vi "Advanced Serial_old.vi"(7 "stop":bool, 8 "read":bool=TRUE, 9 "Write":bool, 11 "string to write":string="*IDN?") -> (0 "RTD-02 (ºC)":sgl format="%0.2f", 1 "RTD-01 (ºC)":sgl format="%0.2f", 2 "vacuo (mBar)":dbl, 3 "P02 (Bar)":dbl, 4 "RTD-chamber (ºC)":sgl format="%0.2f", 5 "P01 (Bar)":dbl, 6 "32bytes":bool)   [LabVIEW 2011]
doc: "The Advanced Serial Read and Write example performs a Serial Port Read, a Serial Port Write, or a combination of these actions while setting some advanced serial features like buffer size, termination characters, and XON/XOFF flow control. The user selects the actions (read or write) on the front panel. If both are selected, the VI will write the data first, read the data and then close the VISA session that is opened to the port. \n\nThe parameters set for the serial port must match the parameters of the connected instrument or device. In this example, the bytes to read parameter specifies the number of bytes that the serial port reads. If there were more bytes at the port than the number specified in bytes to read, those bytes would not be read. Also, if you specify to read more bytes than the number of bytes actually read, you might receive a timeout error message.\n\nINSTRUCTIONS:\n1) Select the serial resource and configuration parameters (baud rate, data bits, parity, stop bits, flow control).\n2) Termination character can be enabled and set. Also, set the required input buffer size prior to running the example.\n3) Select the operations to be performed. \n4) Connect the serial port to your device. If no device is available, perform a loopback test by doing one of the following. Short pins 2 and 3 on a RS-232 cable or short pin 4 to pin 8 and pin 5 to pin 9 on a RS-485/422 cable. \n5) Run the VI to see the data read. (The \"read string\" will match the \"string to write\" if a loopback test was performed.)\n\nThis example exposes several advanced features that you may need for your application. Not all applications need all the features shown in this example. The input buffer size is likely an important setting that you want to control in your application. This example expands upon the flow control option for XON and XOFF, allowing the user to choose those control characters. The timeout parameter has been brought to the front panel so a user can specify the time period the VISA Read will wait for the number of bytes to read before timing out. Also, the user has several controls for the termination character, which is discussed later.\n\nNote that you can press the write and read buttons and change the bytes to read parameters on the fly, while the example is running. However, you must stop the example to change the other configuration parameters after the example has started running, and then run again.\n\nSet the I/O buffer size slightly higher the amount of data you expect to receive. This is very important for applications that don't use flow control, as you may lose characters if the receive buffer overflows.\n\nSetting the timeout period ensures that the operation returns with a timeout error if the operation cannot be performed in the specified time period. \n\nSome devices require a termination character in order to identify the end of command strings. Some devices send a termination character to signify the end of data to be read. \n\nThis example shows how you can end the Read operation once a termination character is detected in the buffer and/or append a termination character at the end of the Write data. To enable the Read to end on a termination character, use the VISA Configure Serial Port or use the VISA Properties Serial End Mode for Reads, Termination Character Enable, and Termination Character. To end the Write with a termination character, use the VISA Properties Serial End Mode for Writes, the Send End Enable, and Termination Character. In this example, the same termination character is used for both the Read and the Write. You can specify two different characters for your application, if desired.\n\nYour application may require specific characters for the XON/XOFF Flow Control. You can specify these characters with the VISA Properties Flow Control XOFF Character and Flow Control XON Character. Note that if the standard XON and XOFF characters are used, then decimal 17 and 19 are unavailable for data values. Remember that using flow control and setting an adequate buffer size allow you to prevent buffer overflows."
uses:
  <vilib>/Instr/_visa.llb/VISA Configure Serial Port (Instr).vi
panel:
  out "actual bytes read":u32
  in  "bytes to read":u32=1000
  out "read string":string
  in  "flow control":u16(ring) items=["None"=0, "XON/XOFF"=1, "RTS/CTS"=2, "DTR/DSR"=4]
  in  "buffer size":u32=4096
  in  "XOFF Character":u8=19 format="%.0x"
  in  "XON Character":u8=17 format="%.0x"
  in  "termination char\n(0xA = '\\n' = LF)":u8=10 format="%.0x"
  in  "timeout (ms)":u32=10000
  in  "parity":u16(ring) items=["None", "Odd", "Even", "Mark", "Space"]
  in  "data bits":u16=8 min=5 max=8 step=1
  in  "stop bits":u16(ring)=10 items=["1.0"=10, "1.5"=15, "2.0"=20]
  out "baud rate":u32=9600
  in  "VISA resource name":refnum<visa-resource-name>="COM1"
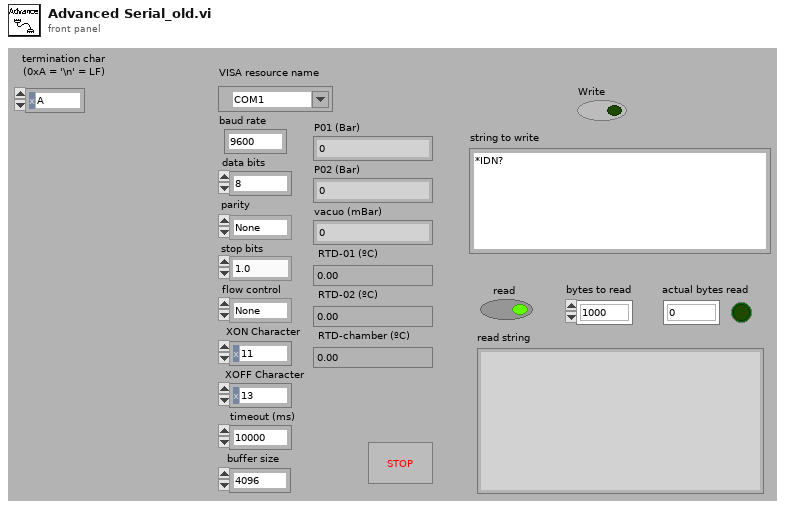
[diagram p1: front panel]
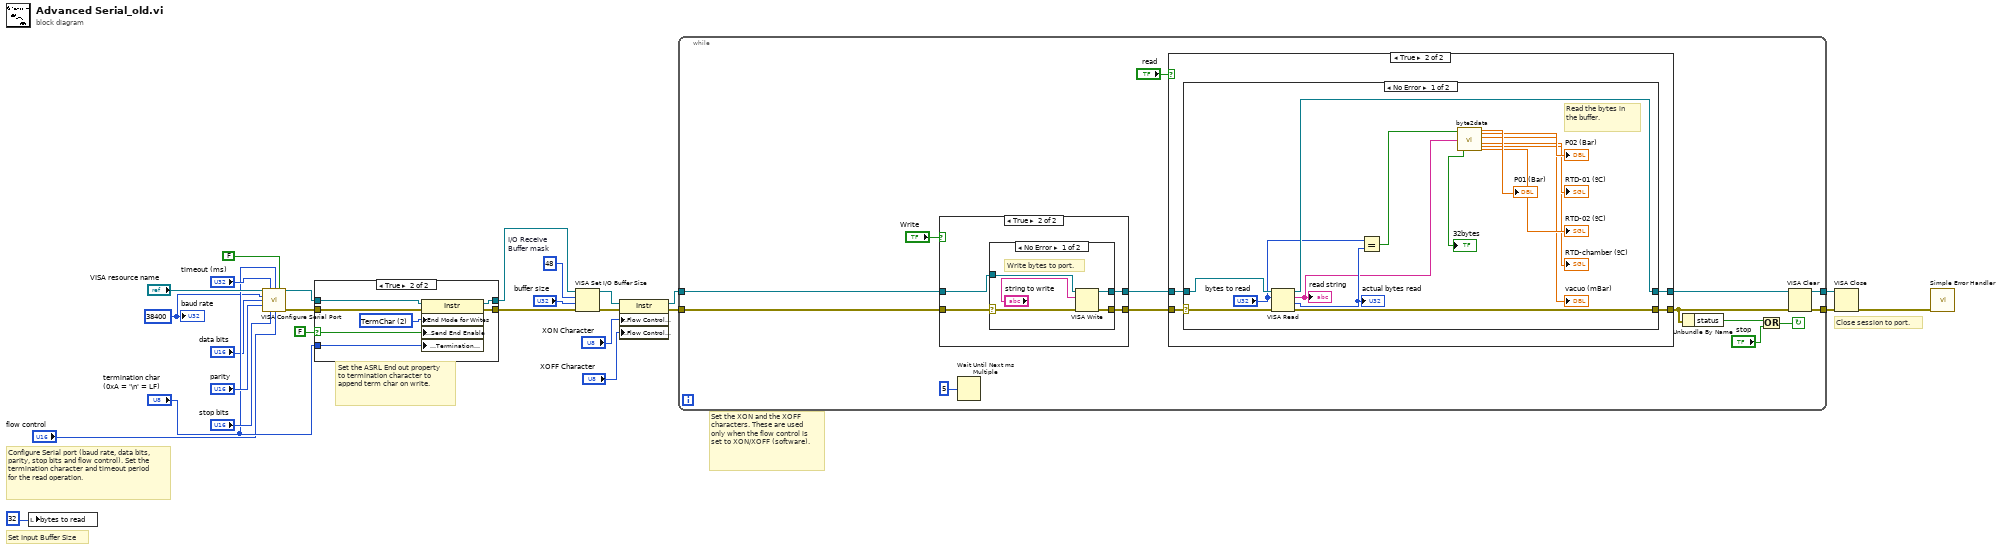
[diagram p0: block diagram]
diagram:
  w2 = u32 38400 ("baud rate 2")
  w20 = u16 48  # I/O Receive Buffer mask
  # "Set the XON and the XOFF characters. These are used only when the flow control is set to XON/XOFF (software)."
  # "Configure Serial port (baud rate, data bits, parity, stop bits and flow control). Set the termination character and timeout period for the read operation."
  # "Set Input Buffer Size"
  # "Set the ASRL End out property to termination character to append term char on write."
  # "Close session to port."
  n1 = local write "bytes to read"(u32 32 ("bytes to read")) -> ()
  n2 = call-poly "VISA Configure Serial Port"("VISA resource name"="VISA resource name", "timeout (10sec)"="timeout (ms)", "termination char\n(0xA = '\\n' = LF)"="termination char\n(0xA = '\\n' = LF)", "Enable Termination\nChar (T)"=FALSE ("End read on termination character?"), "baud rate (9600)"=w2, "data bits (8)"="data bits", "parity (0:none)"="parity", "stop bits (10: 1 bit)"="stop bits", "flow control (0:none)"="flow control") -> ("VISA resource name out"=w6:refnum<visa-resource-name>, "error out"=w9:errorcluster)  [unwired: 1 in, 4 out]
  n3 = case shown="True" FALSE ("End write with termination character?") {
    selector: FALSE ("End write with termination character?") -> [_ w29]
    tunnel: w6 -> [w27 w35]
    tunnel: w9 -> [w28 w34]
    tunnel: [w27 w33] -> w7
    tunnel: [w28 w32] -> w8
    tunnel: "termination char\n(0xA = '\\n' = LF)" -> [_ w30]
    frame False {
    }
    frame True {
      w31 = u16 2 items=["None", "LastBit", "TermChar", "Break"] ("Serial Settings:Serial End Mode for Writes")
      n4 = property class="Instr"(reference=w35, error in=w34, "Serial Settings:End Mode for Writes"=w31, "Message Based Settings:Send End Enable"=w29, "Message Based Settings:Termination Character"=w30) -> (reference out=w33:refnum<visa-resource-name>, error out=w32:errorcluster)
    }
  }
  n5 = VISA Set I/O Buffer Size(VISA resource name=w7, mask (16)=w20, size (4096)="buffer size", error in (no error)=w8) -> (VISA resource name out=w15:refnum<visa-resource-name>, error out=w14:errorcluster)
  n6 = property class="Instr"(reference=w15, error in=w14, "Serial Settings:Flow Control XON Character"="XON Character", "Serial Settings:Flow Control XOFF Character"="XOFF Character") -> (reference out=w5:refnum<visa-resource-name>, error out=w11:errorcluster)
  n7 = while {
    tunnel: w11 -> [w43]
    tunnel: w5 -> [w44]
    tunnel: [w37] -> w4
    tunnel: [w36] -> w3
    stop <- w42 continue-if-true
    n8 = case shown="True" "Write" {
      tunnel: [w51 w55] -> w46
      tunnel: [w50 w54] -> w45
      tunnel: w44 -> [w51 w53]
      tunnel: w43 -> [w50 w52]
      frame False {
      }
      frame True {
        n9 = case shown="No Error" w52 {
          selector: w52 -> [w57 w62]
          tunnel: [w60 w61] -> w55
          tunnel: [w59 w62] -> w54
          tunnel: w53 -> [w58 w61]
          frame No Error {
            # "Write bytes to port."
            n10 = VISA Write(VISA resource name=w58, write buffer="string to write", error in (no error)=w57) -> (VISA resource name out=w60:refnum<visa-resource-name>, error out=w59:errorcluster)  [unwired: 1 out]
          }
          frame Error {
          }
        }
      }
    }
    n11 = Wait Until Next ms Multiple(millisecond multiple=u32 5) -> ()  [unwired: 1 out]
    n12 = case shown="True" "read" {
      tunnel: w45 -> [w63 w66]
      tunnel: w46 -> [w64 w65]
      tunnel: [w63 w68] -> w39
      tunnel: [w64 w67] -> w38
      frame False {
      }
      frame True {
        n13 = case "Read bytes from port." shown="No Error" w66 {
          selector: w66 -> [w80 w84]
          tunnel: [w82 w84] -> w68
          tunnel: [w83 w85] -> w67
          tunnel: w65 -> [w81 w85]
          frame No Error {
            # "Read the bytes in the buffer."
            n14 = VISA Read(VISA resource name=w81, byte count="bytes to read", error in (no error)=w80) -> (VISA resource name out=w83:refnum<visa-resource-name>, read buffer=w76:string, return count=w78:u32, error out=w82:errorcluster)
            "read string" <- w76
            "actual bytes read" <- w78
            n15 = Equal?(x="bytes to read", y=w78) -> (x = y?=w77:bool)
            n16 = call "byte2data.vi"("string"=w76, "Read"=w77) -> ("RTD-02 (ºC)"=→"RTD-02 (ºC)":sgl, "RTD-chamber (ºC)"=→"RTD-chamber (ºC)":sgl, "RTD-01 (ºC)"=→"RTD-01 (ºC)":sgl, "P02 (Bar)"=→"P02 (Bar)":dbl, "vacuo (mBar)"=→"vacuo (mBar)":dbl, "P01 (Bar)"=→"P01 (Bar)":dbl, "OK"=→"32bytes":bool)
          }
          frame Error {
            # "Error occurred \nreading Bytes at \nSerial Port"
          }
        }
      }
    }
    n17 = Unbundle By Name(w39) -> ("status"=w47:bool)
    n18 = Or(x=w47, y="stop") -> (x .or. y?=w42:bool)
    n19 = VISA Clear(VISA resource name=w38, error in (no error)=w39) -> (VISA resource name out=w37:refnum<visa-resource-name>, error out=w36:errorcluster)
  }
  n20 = VISA Close(VISA resource name=w4, error in (no error)=w3) -> (error out=w25:errorcluster)
  n21 = call <vilib>:"Simple Error Handler.vi"("error in (no error)"=w25) -> ()  [unwired: 1 in, 8 out]
  "baud rate" <- w2
